vi "CalculoTestePontos_Validacao.vi"(10 "TempoEntrePontos":dbl, 11 "Pontos":dbl[](array[numeric])) -> (3 "XY Graph":cluster{"X":dbl, "Y":dbl}[](graph))   [LabVIEW 2019]
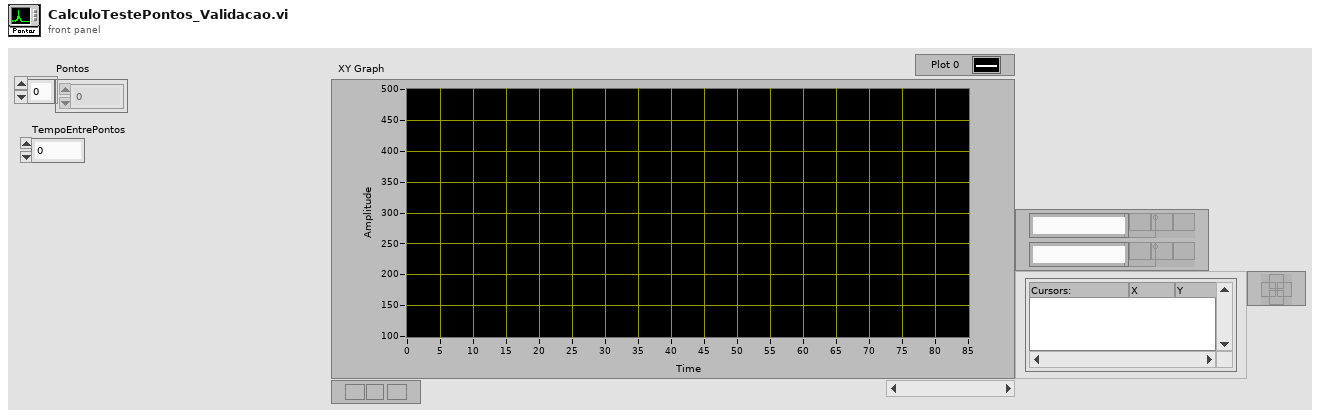
[diagram p1: front panel]
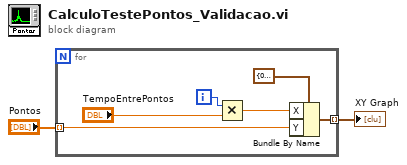
[diagram p0: block diagram]
diagram:
  n1 = for {
    tunnel: "Pontos" -> [w7] mode=indexing
    tunnel: [w3] -> w1 mode=indexing
    i -> [w5]
    n2 = Multiply(x=w5, y="TempoEntrePontos") -> (x*y=w4:dbl)
    n3 = Bundle By Name(cluster=cluster{"X":dbl, "Y":dbl} {"X"=0.0, "Y"=0.0} ("new element/subarray"), "X"=w4, "Y"=w7) -> (w3:cluster{"X":dbl, "Y":dbl})
  }
  "XY Graph" <- w1
